vi "Get_Latest_id_dust_event.vi"(8 "error in (no error)":errorcluster, 11 "Small?":bool) -> (0 "error out":errorcluster, 3 "id_dust_event":i64)   [LabVIEW 2013]
uses:
  <vilib>/addons/database/Connection.llb/Conn Execute.vi
  <vilib>/addons/database/Recordset.llb/Rec Fetch Recordset Data (R).vi
  <vilib>/addons/database/Recordset.llb/Rec Destroy - Connection.vi
  <vilib>/addons/database/_DB Variant To Data/Database Variant To Data.xnode
  <vilib>/addons/database/NI_Database_API.lvlib
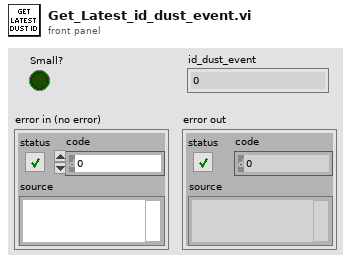
[diagram p1: front panel]
types:
  T1 = typedef "NI_Database_API.lvlib/Conn ObjectReference.ctl" = refnum<k1>
  T2 = typedef "NI_Database_API.lvlib/Rec ObjectReference.ctl" = refnum<k1>
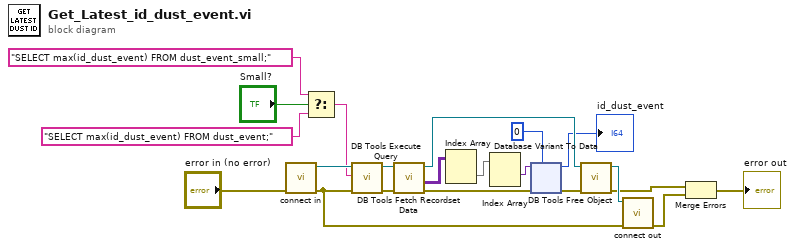
[diagram p0: block diagram]
diagram:
  n1 = call "connect in.vi"("error in (no error)"="error in (no error)") -> ("error out"=w20:errorcluster, "Database Connection"=w21:T1)  [unwired: 6 in, 1 out]
  n2 = Select(t="SELECT max(id_dust_event) FROM dust_event_small;" ("SQL query"), s="Small?", f="SELECT max(id_dust_event) FROM dust_event;" ("SQL query")) -> (s? t:f=w1:string)
  n3 = call-poly <vilib>:"DB Tools Execute Query.vi"("error in (no error)"=w20, "SQL query"=w1, "connection reference"=w21) -> ("error out"=w14:errorcluster, "recordset reference"=w13:T2)  [unwired: 5 in]
  n4 = call-poly <vilib>:"DB Tools Fetch Recordset Data.vi"("error in (no error)"=w14, "recordset reference"=w13) -> ("error out"=w17:errorcluster, "recordset data"=w15:variant[][], "recordset reference out"=w8:T2)  [unwired: 3 in]
  n5 = Index Array(array=w15) -> (element=w19:variant[])  [unwired: 2 in]
  n6 = Index Array(array=w19) -> (element #1=w18:variant)  [unwired: 2 in, 1 out]
  n7 = xnode "Database Variant To Data"("database variant"=w18, "error in (no error)"=w17, "type"=0) -> ("data"=→"id_dust_event":i32, "error out"=w12:errorcluster)
  n8 = call-poly <vilib>:"DB Tools Free Object.vi"("error in (no error)"=w12, "recordset reference"=w8) -> ("error out"=w9:errorcluster, "connection reference"=w11:T1)  [unwired: 8 in]
  n9 = call "connect out.vi"("error in (no error)"=w20, "connection reference"=w11) -> ("error out"=w10:errorcluster)  [unwired: 9 in]
  n10 = Merge Errors(w9, w10) -> (→"error out":errorcluster)
